vi "Collect waveforms.vi"(6 "max len":i32, 7 "init":bool, 11 "waveforms":waveform(dbl)[](array[waveform])) -> (3 "waveforms out":waveform(dbl)[](array[waveform]))   [LabVIEW 2012]
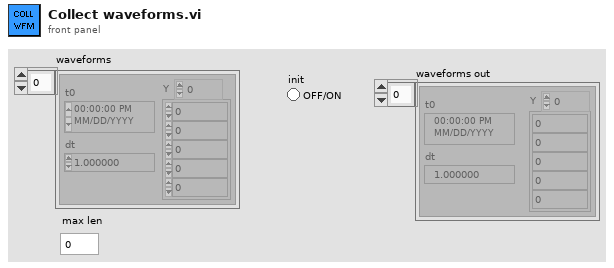
[diagram p1: front panel]
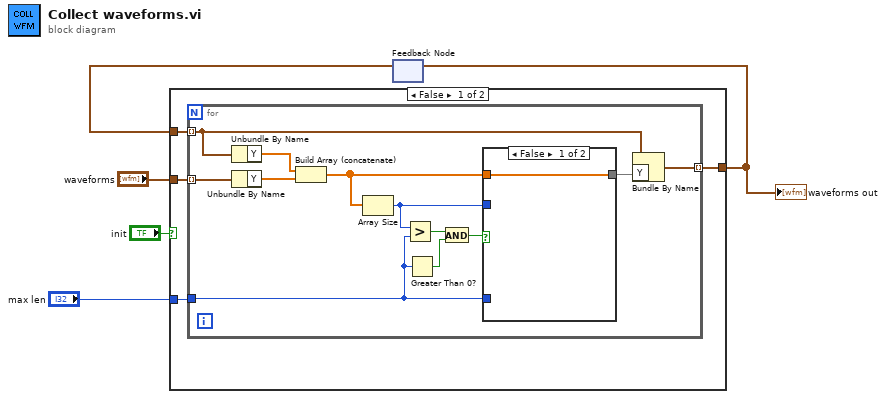
[diagram p0: block diagram]
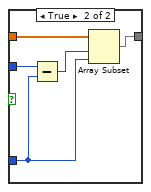
[diagram p2: hidden frame]
diagram:
  n1 = feedback #1() -> (w2:waveform(dbl)[])  [unwired: 1 in]
  n2 = case shown="False" "init" {
    tunnel: "waveforms" -> [w9 w28]
    tunnel: "max len" -> [w8 _]
    tunnel: [w7 w28] -> w3
    tunnel: w2 -> [w6 _]
    frame False {
      n3 = for {
        tunnel: w9 -> [w21] mode=indexing
        tunnel: w6 -> [w12] mode=indexing
        tunnel: w8 -> [w13]
        tunnel: [w10] -> w7 mode=indexing
        n4 = Unbundle By Name(w12) -> ("Y"=w19:dbl[])
        n5 = Unbundle By Name(w21) -> ("Y"=w20:dbl[])
        n6 = Build Array (concatenate)(w19, w20) -> (w18:dbl[])
        n7 = Array Size(array=w18) -> (size(s)=w14:i32)
        n8 = Greater?(x=w14, y=w13) -> (0:w17:bool)
        n9 = Greater Than 0?(x=w13) -> (x > 0?=w16:bool)
        n10 = And(x=w17, y=w16) -> (x .and. y?=w15:bool)
        n11 = case shown="False" w15 {
          tunnel: w18 -> [w22 w27]
          tunnel: w14 -> [_ w26]
          tunnel: w13 -> [_ w24]
          tunnel: [w22 w23] -> w11
          frame False {
          }
          frame True {
            n12 = Subtract(x=w26, y=w24) -> (x-y=w25:i32)
            n13 = Array Subset(array=w27, index=w25, length=w24) -> (w23:dbl[])
          }
        }
        n14 = Bundle By Name(cluster=w12, "Y"=w11) -> (w10:waveform(dbl))
      }
    }
    frame True {
    }
  }
  "waveforms out" <- w3
  n15 = feedback-in #1(w3) -> ()
